vi "testAssertionFailureMessage.vi"() -> ()   [LabVIEW 2019, in "AssertionTest.lvlib" / "AssertNoError.lvlib"]
uses:
  AssertNoError.lvlib
  <vilib>/Utility/error.llb/Error Cluster From Error Code.vi
  <vilib>/ErrorRing/Error Ring.xnode
  Assertion/Assertion.lvlib
  AssertionTest.lvlib
panel:
  out "error out":errorcluster
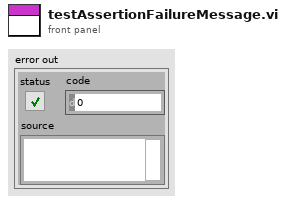
[diagram p1: front panel]
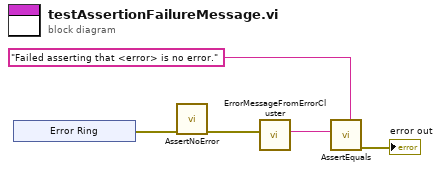
[diagram p0: block diagram]
diagram:
  n1 = xnode "Error Ring"() -> ("error out"=w5:errorcluster)
  n2 = call "AssertNoError.vi"("error in (no error)"=w5) -> ("error out"=w3:errorcluster)  [unwired: 10 in]
  n3 = call "ErrorMessageFromErrorCluster.vi"("Error"=w3) -> ("Error Message"=w2:string)  [unwired: 10 in]
  n4 = call "AssertEquals.vi"("Expected"="Failed asserting that <error> is no error." ("Needle"), "Actual"=w2) -> ("error out"=→"error out":errorcluster)  [unwired: 9 in]
